vi "ChangeExistingname(SubVI).vi"(10 "Numb":i32, 11 "Name In":string) -> (2 "Result string":string)   [LabVIEW 2018]
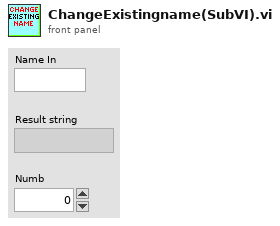
[diagram p1: front panel]
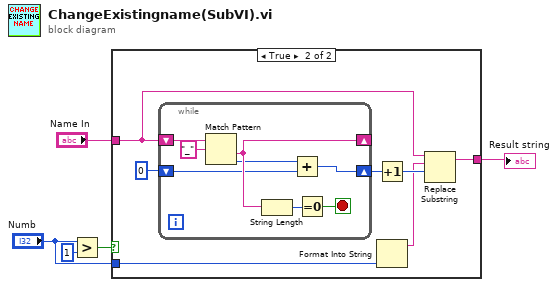
[diagram p0: block diagram]
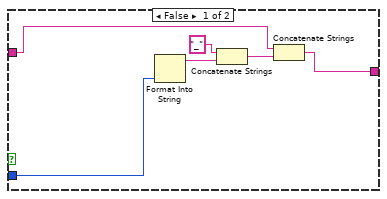
[diagram p2: hidden frame]
diagram:
  n1 = Greater?(x="Numb", y=1) -> (0:w5:bool)
  n2 = case shown="True" w5 {
    tunnel: "Numb" -> [w8 w14]
    tunnel: [w6 w13] -> w4
    tunnel: "Name In" -> [w7 w12]
    frame False {
      n3 = Format Into String(w8) -> (resulting string=w10:string)  [unwired: 3 in, 1 out]
      n4 = Concatenate Strings("_" ("string"), w10) -> (w11:string)
      n5 = Concatenate Strings(w7, w11) -> (w6:string)
    }
    frame True {
      n6 = while {
        shift-right: [w22] -> _
        shift-left: w12 -> [w26]
        shift-right: [w19] -> w17
        shift-left: 0 ("offset past match") -> [w20]
        stop <- w23 stop-if-true
        n7 = Match Pattern(string=w26, regular expression="_") -> (after substring=w22:string, offset past match=w21:i32)  [unwired: 1 in, 2 out]
        n8 = String Length(string=w22) -> (length=w24:i32)
        n9 = Add(x=w21, y=w20) -> (x+y=w19:i32)
        n10 = Equal To 0?(x=w24) -> (x = 0?=w23:bool)
      }
      n11 = Increment(x=w17) -> (x+1=w16:i32)
      n12 = Format Into String(w14) -> (resulting string=w15:string)  [unwired: 3 in, 1 out]
      n13 = Replace Substring(3:w16, 4:w15, 5:w12) -> (1:w13:string)  [unwired: 1 in, 1 out]
    }
  }
  "Result string" <- w4
